vi "EPIC_AI Main.vi"() -> ()   [LabVIEW 2014]
uses:
  <vilib>/DAQmx/read.llb/DAQmx Read (Analog 2D DBL NChan NSamp).vi
panel:
  out "Ch 2":waveform(dbl)(graph)
  out "Ch 1":waveform(dbl)(graph)
  in  "Scale":cluster{"Ch 1":dbl, "Ch 2":dbl}={"Ch 1"=1.0, "Ch 2"=1.0} {"Ch 2" format="%#.6f"; "Ch 1" format="%#.6f"}
  out "AI 1,2":waveform(dbl)[](graph)
  out "1-2":waveform(dbl)(graph)
  in  "정지":bool
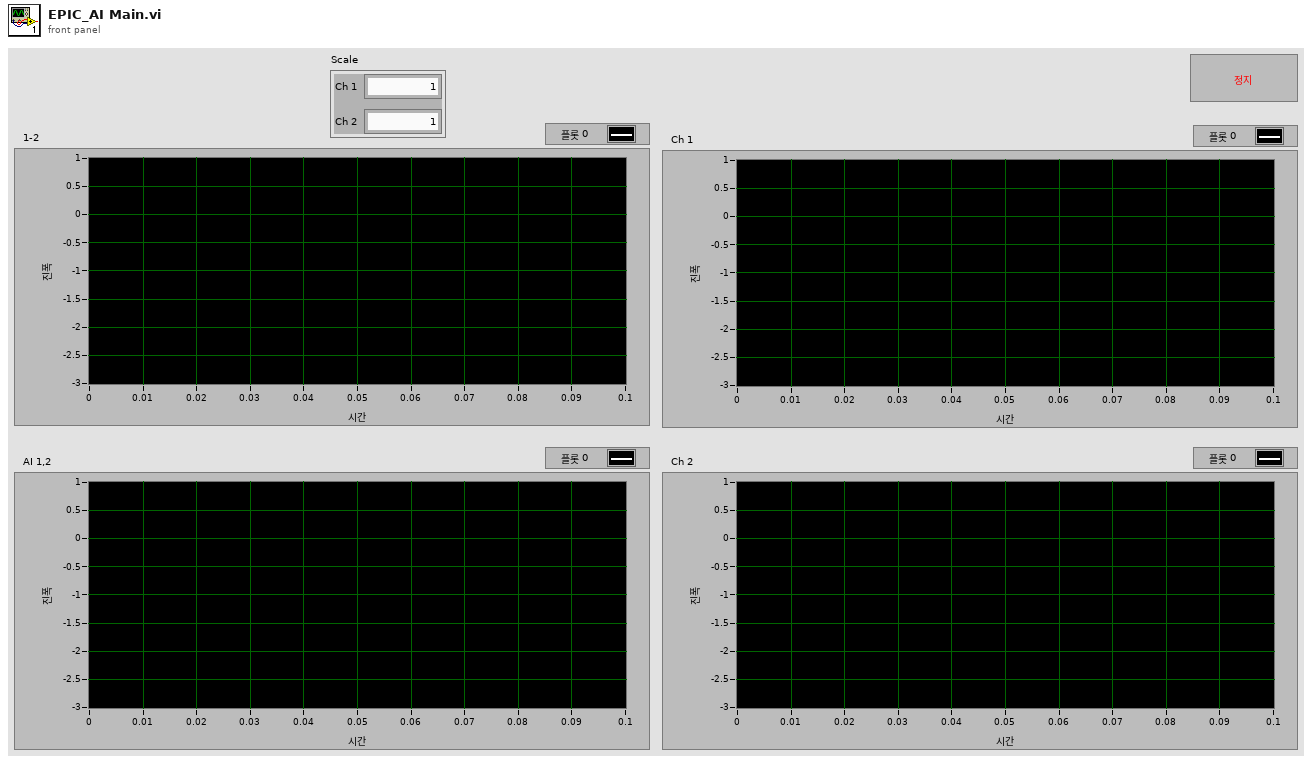
[diagram p1: front panel]
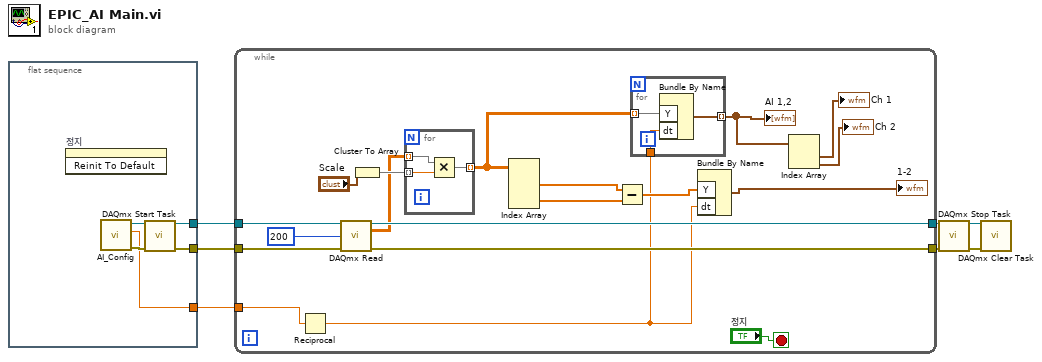
[diagram p0: block diagram]
diagram:
  n1 = flat-sequence {
    tunnel: [w10] -> w7
    tunnel: [w9] -> w6
    tunnel: [w8] -> w1
    frame #0 {
      n2 = invoke on="정지" class="Bool" method="Reinit To Default"() -> ()  [unwired: 3 in, 3 out]
      n3 = call "AI_Config.vi"() -> ("error out"=w11:errorcluster, "rate"=w8:dbl, "task out"=w12:refnum<k21>)  [unwired: 9 in]
      n4 = call <vilib>:"DAQmx Start Task.vi"("task/channels in"=w12, "error in"=w11) -> ("task out"=w9:refnum<k21>, "error out"=w10:errorcluster)  [unwired: 12 in]
    }
  }
  n5 = while {
    tunnel: w7 -> [w30]
    tunnel: w6 -> [w29]
    tunnel: [w27] -> w3
    tunnel: [w26] -> w2
    tunnel: w1 -> [w22]
    stop <- "정지" stop-if-true
    n6 = Reciprocal(x=w22) -> (1/x=w20:dbl)
    n7 = call-poly <vilib>:"DAQmx Read.vi"("task/channels in"=w29, "number of samples per channel"=200, "error in"=w30) -> ("task out"=w27:refnum<k21>, "data"=w17:dbl[][], "error out"=w26:errorcluster)  [unwired: 10 in]
    n8 = Cluster To Array(cluster="Scale") -> (array=w18:dbl[])
    n9 = for {
      tunnel: w17 -> [w34] mode=indexing
      tunnel: w18 -> [w33] mode=indexing
      tunnel: [w32] -> w16 mode=indexing
      n10 = Multiply(x=w34, y=w33) -> (x*y=w32:dbl[])
    }
    n11 = Index Array(array=w16) -> (element #1=w25:dbl[], element #2=w24:dbl[])  [unwired: 4 in]
    n12 = Subtract(x=w25, y=w24) -> (x-y=w23:dbl[])
    n13 = for {
      tunnel: w20 -> [w37]
      tunnel: w16 -> [w36] mode=indexing
      tunnel: [w35] -> w15 mode=indexing
      n14 = Bundle By Name("Y"=w36, "dt"=w37) -> (w35:waveform(dbl))  [unwired: 1 in]
    }
    "AI 1,2" <- w15
    n15 = Bundle By Name("Y"=w23, "dt"=w20) -> (→"1-2":waveform(dbl))  [unwired: 1 in]
    n16 = Index Array(array=w15) -> (element #1=→"Ch 1":waveform(dbl), element #2=→"Ch 2":waveform(dbl))  [unwired: 2 in]
  }
  n17 = call <vilib>:"DAQmx Stop Task.vi"("task/channels in"=w3, "error in"=w2) -> ("task out"=w5:refnum<k21>, "error out"=w4:errorcluster)  [unwired: 12 in]
  n18 = call <vilib>:"DAQmx Clear Task.vi"("task in"=w5, "error in"=w4) -> ()  [unwired: 13 in, 1 out]
